vi "Arduino_comm.vi"() -> ()   [LabVIEW 2018]
panel:
  out "concatenated string":string
  out "VISA resource name out":refnum<visa-resource-name>
  out "error out 2":errorcluster
  in  "baud rate (115200)":u32=115200
  in  "VISA resource name":refnum<visa-resource-name>
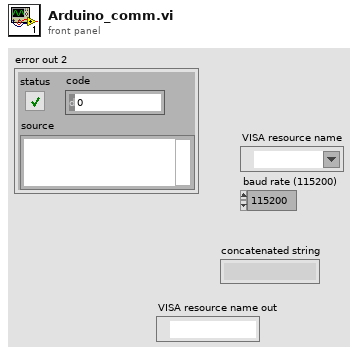
[diagram p1: front panel]
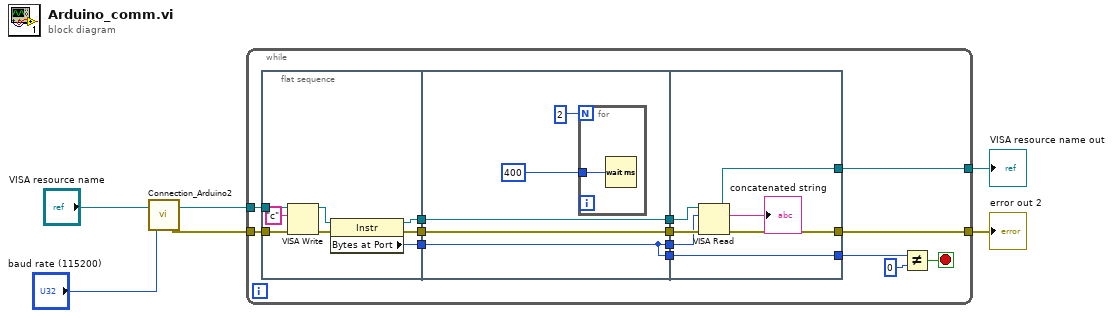
[diagram p0: block diagram]
diagram:
  n1 = call "Connection_Arduino2.vi"("baud rate (9600)"="baud rate (115200)", "VISA resource name"="VISA resource name") -> ("error out"=w1:errorcluster, "VISA resource name out"=w2:refnum<visa-resource-name>)
  n2 = while {
    tunnel: [w13] -> w4
    tunnel: [w12] -> w3
    tunnel: w2 -> [w8]
    tunnel: w1 -> [w7]
    stop <- w9 stop-if-true
    n3 = flat-sequence {
      tunnel: [w26] -> w20
      tunnel: [w25] -> w19
      tunnel: [w24] -> w18
      tunnel: w8 -> [w23]
      tunnel: w7 -> [w22]
      tunnel: w20 -> [w32]
      tunnel: [w32] -> w17
      tunnel: [w31] -> w16
      tunnel: w19 -> [w31]
      tunnel: [w30] -> w15
      tunnel: w18 -> [w30]
      tunnel: [w30] -> w11
      tunnel: w17 -> [w37]
      tunnel: w16 -> [w36]
      tunnel: w15 -> [w38]
      tunnel: [w40] -> w12
      tunnel: [w39] -> w13
      tunnel: [w38] -> w10
      tunnel: w11 -> [w35]
      frame #0 {
        n4 = VISA Write(VISA resource name=w23, write buffer="c", error in (no error)=w22) -> (VISA resource name out=w28:refnum<visa-resource-name>, error out=w27:errorcluster)  [unwired: 1 out]
        n5 = property class="Instr"(reference=w28, error in=w27) -> (reference out=w26:refnum<visa-resource-name>, error out=w25:errorcluster, "Bytes at Port"=w24:u32)
      }
      frame #1 {
        n6 = for {
          N: 2 -> [_]
          tunnel: u32 400 ("milliseconds to wait") -> [w34]
          n7 = Wait (ms)(milliseconds to wait=w34) -> ()  [unwired: 1 out]
        }
      }
      frame #2 {
        n8 = VISA Read(VISA resource name=w37, byte count=w35, error in (no error)=w36) -> (VISA resource name out=w40:refnum<visa-resource-name>, read buffer=→"concatenated string":string, error out=w39:errorcluster)  [unwired: 1 out]
      }
    }
    n9 = Not Equal?(x=w10, y=0) -> (x != y?=w9:bool)
  }
  "error out 2" <- w4
  "VISA resource name out" <- w3
